vi "ExX4CamerasSameGraph.vi"() -> ()   [LabVIEW 2010]
panel:
  out "Camera 16":sgl[](graph)
  out "Camera 15":sgl[](graph)
  out "Camera 14":sgl[](graph)
  out "Camera 13":sgl[](graph)
  out "Camera 12":sgl[](graph)
  out "Camera 11":sgl[](graph)
  out "Camera 10":sgl[](graph)
  out "Camera 9":sgl[](graph)
  out "Camera 8":sgl[](graph)
  out "Camera 7":sgl[](graph)
  out "Camera 6":sgl[](graph)
  out "Camera 5":sgl[](graph)
  out "Camera 4":sgl[](graph)
  out "Camera 3":sgl[](graph)
  out "Camera 2":sgl[](graph)
  out "Camera 1":sgl[](graph)
  in  "stop":bool
  in  "Exposure":dbl=0.5 format="%.2f"
  out "error out":errorcluster
  in  "error in (no error)":errorcluster
  # "Ex2CamerasSameGraph:\nThis example runs two cameras in focus mode.\nSets them up for center strip and displays as graph.\nRemember to setup two cameras in the pvcam.ini\nfile."
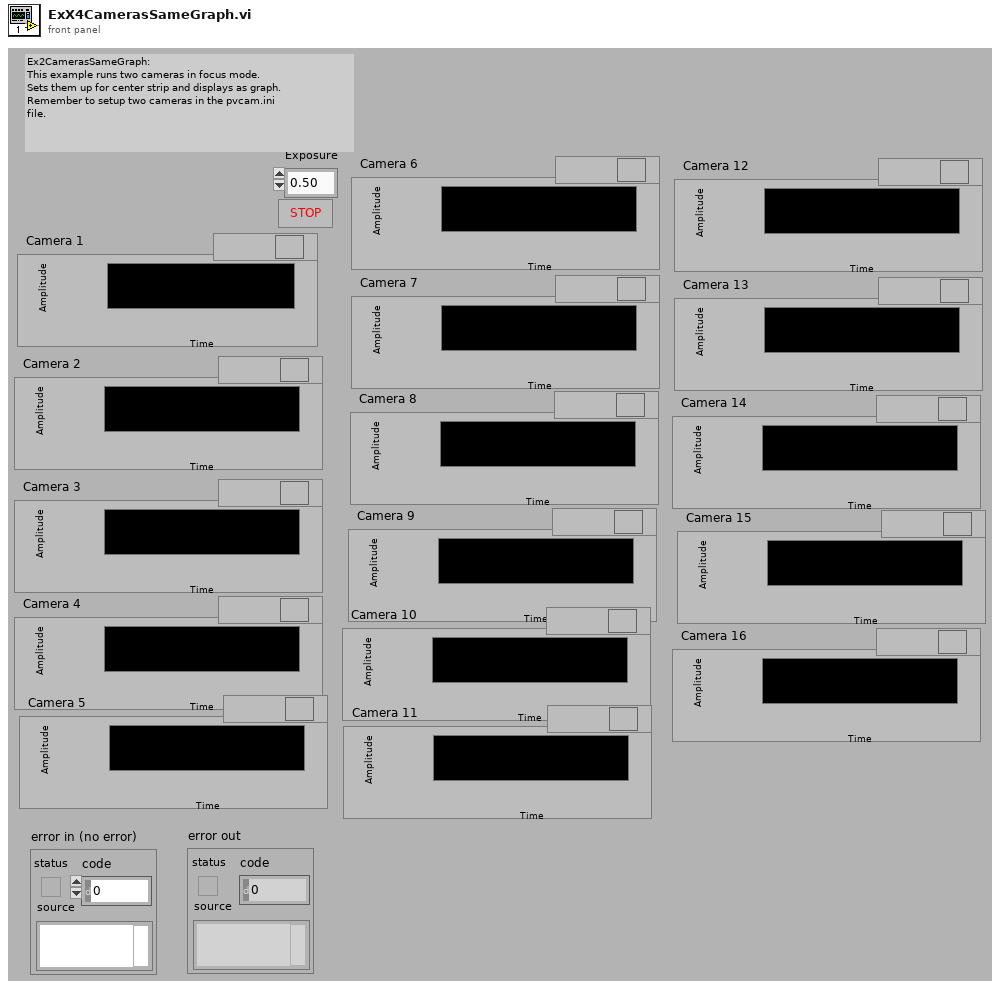
[diagram p1: front panel]
types:
  T1 = cluster{"Camera Handle":u32, "Camera Handle":u32, "Camera Handle":u32, "Camera Handle":u32}
  T2 = cluster{"Image Handle":u32, "Image Handle":u32, "Image Handle":u32, "Image Handle":u32}
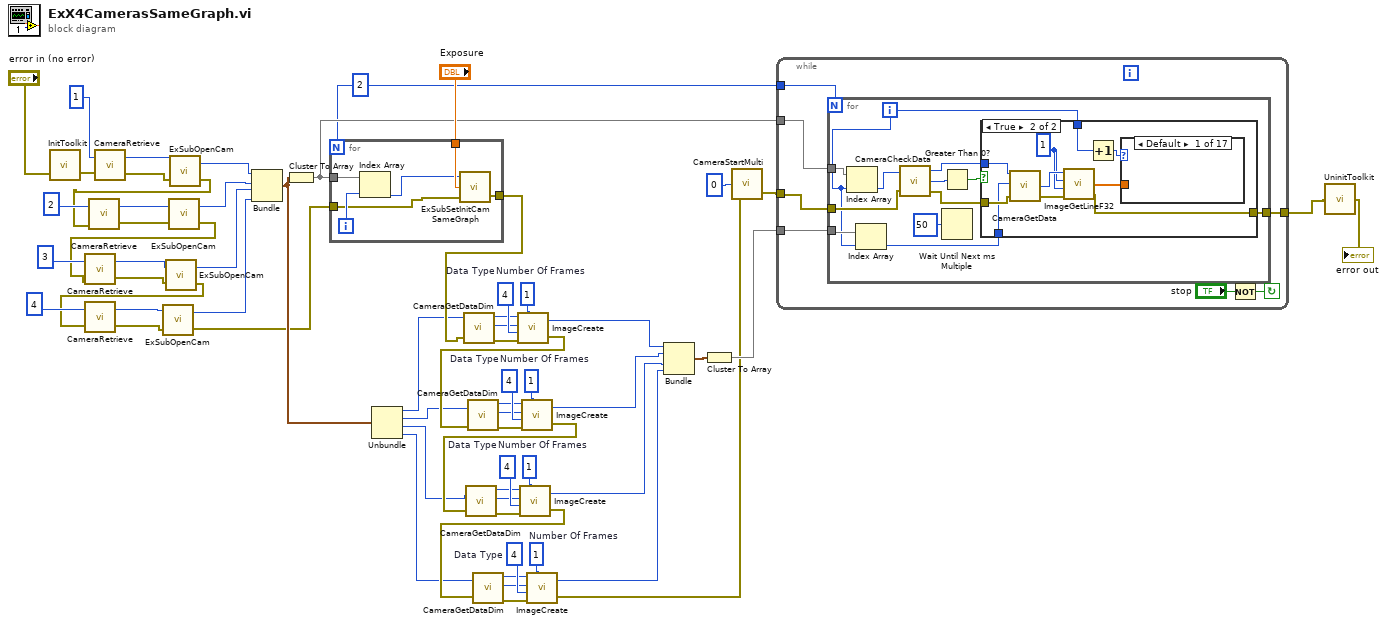
[diagram p0: block diagram]
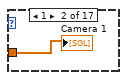
[diagram p3: hidden frame]
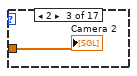
[diagram p4: hidden frame]
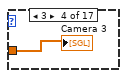
[diagram p5: hidden frame]
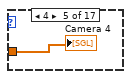
[diagram p6: hidden frame]
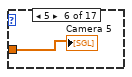
[diagram p7: hidden frame]
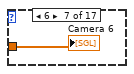
[diagram p8: hidden frame]
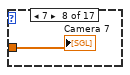
[diagram p9: hidden frame]
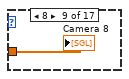
[diagram p10: hidden frame]
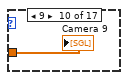
[diagram p11: hidden frame]
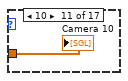
[diagram p12: hidden frame]
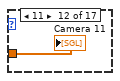
[diagram p13: hidden frame]
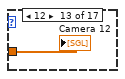
[diagram p14: hidden frame]
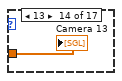
[diagram p15: hidden frame]
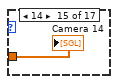
[diagram p16: hidden frame]
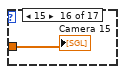
[diagram p17: hidden frame]
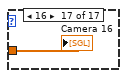
[diagram p18: hidden frame]
diagram:
  w37 = u32 1  # Number Of Frames
  w38 = u32 4  # Data Type
  w42 = u32 1  # Number Of Frames
  w43 = u32 4  # Data Type
  w47 = u32 1  # Number Of Frames
  w48 = u32 4  # Data Type
  w52 = u32 1  # Number Of Frames
  w53 = u32 4  # Data Type
  w55 = 2
  n1 = call <userlib>:"InitToolkit.vi"("error in"="error in (no error)") -> ("error out"=w64:errorcluster)
  n2 = call <userlib>:"CameraRetrieve.vi"("error in"=w64, "Camera Index"=1) -> ("error out"=w7:errorcluster, "Device ID"=w8:u32)
  n3 = call "ExSubOpenCam.vi"("error in (no error)"=w7, "Camera Device ID"=w8) -> ("error out"=w6:errorcluster, "Camera Handle"=w9:u32)
  n4 = call <userlib>:"CameraRetrieve.vi"("error in"=w6, "Camera Index"=2) -> ("error out"=w5:errorcluster, "Device ID"=w14:u32)
  n5 = call "ExSubOpenCam.vi"("error in (no error)"=w5, "Camera Device ID"=w14) -> ("error out"=w4:errorcluster, "Camera Handle"=w10:u32)
  n6 = call <userlib>:"CameraRetrieve.vi"("error in"=w4, "Camera Index"=3) -> ("error out"=w34:errorcluster, "Device ID"=w31:u32)
  n7 = call "ExSubOpenCam.vi"("error in (no error)"=w34, "Camera Device ID"=w31) -> ("error out"=w3:errorcluster, "Camera Handle"=w11:u32)
  n8 = call <userlib>:"CameraRetrieve.vi"("error in"=w3, "Camera Index"=4) -> ("error out"=w1:errorcluster, "Device ID"=w2:u32)
  n9 = call "ExSubOpenCam.vi"("error in (no error)"=w1, "Camera Device ID"=w2) -> ("error out"=w13:errorcluster, "Camera Handle"=w12:u32)
  n10 = Bundle("Camera Handle"=w9, "Camera Handle"=w10, "Camera Handle"=w11, "Camera Handle"=w12) -> (w19:T1)  [unwired: 1 in]
  n11 = Cluster To Array(cluster=w19) -> (array=w58:u32[])
  n12 = for {
    N: w55 -> [_]
    tunnel: w58 -> [w71]
    tunnel: w13 -> [w67]
    tunnel: [w69] -> w24
    tunnel: "Exposure" -> [w68]
    i -> [w70]
    n13 = Index Array(array=w71, index=w70) -> (element=w66:u32)
    n14 = call "ExSubSetInitCamSameGraph.vi"("error in (no error)"=w67, "Exposure"=w68, "Camera Handle"=w66) -> ("error out"=w69:errorcluster)  [unwired: 1 out]
  }
  n15 = Unbundle(w19) -> ("Camera Handle"=w18:u32, "Camera Handle"=w17:u32, "Camera Handle"=w16:u32, "Camera Handle"=w15:u32)
  n16 = call <userlib>:"CameraGetDataDim.vi"("Camera Handle"=w18, "error in"=w24) -> ("Xdim"=w50:u32, "Ydim"=w51:u32, "error out"=w54:errorcluster)  [unwired: 1 out]
  n17 = call <userlib>:"ImageCreate.vi"("X dimension"=w50, "Y dimension"=w51, "Data Type"=w53, "error in"=w54, "Number Of Frames"=w52) -> ("Image Handle"=w30:u32, "error out"=w23:errorcluster)
  n18 = call <userlib>:"CameraGetDataDim.vi"("Camera Handle"=w17, "error in"=w23) -> ("Xdim"=w45:u32, "Ydim"=w46:u32, "error out"=w49:errorcluster)  [unwired: 1 out]
  n19 = call <userlib>:"ImageCreate.vi"("X dimension"=w45, "Y dimension"=w46, "Data Type"=w48, "error in"=w49, "Number Of Frames"=w47) -> ("Image Handle"=w29:u32, "error out"=w22:errorcluster)
  n20 = call <userlib>:"CameraGetDataDim.vi"("Camera Handle"=w16, "error in"=w22) -> ("Xdim"=w40:u32, "Ydim"=w41:u32, "error out"=w44:errorcluster)  [unwired: 1 out]
  n21 = call <userlib>:"ImageCreate.vi"("X dimension"=w40, "Y dimension"=w41, "Data Type"=w43, "error in"=w44, "Number Of Frames"=w42) -> ("Image Handle"=w28:u32, "error out"=w21:errorcluster)
  n22 = call <userlib>:"CameraGetDataDim.vi"("Camera Handle"=w15, "error in"=w21) -> ("Xdim"=w35:u32, "Ydim"=w36:u32, "error out"=w39:errorcluster)  [unwired: 1 out]
  n23 = call <userlib>:"ImageCreate.vi"("X dimension"=w35, "Y dimension"=w36, "Data Type"=w38, "error in"=w39, "Number Of Frames"=w37) -> ("Image Handle"=w27:u32, "error out"=w20:errorcluster)
  n24 = Bundle("Image Handle"=w30, "Image Handle"=w29, "Image Handle"=w28, "Image Handle"=w27) -> (w26:T2)  [unwired: 1 in]
  n25 = Cluster To Array(cluster=w26) -> (array=w25:u32[])
  n26 = call "CameraStartMulti.vi"("error in (no error)"=w20, "Number Of Cameras"=0) -> ("error out"=w60:errorcluster)  [unwired: 1 in, 1 out]
  n27 = while {
    tunnel: w60 -> [w75]
    tunnel: w58 -> [w76]
    tunnel: [w74] -> w56
    tunnel: w55 -> [w73]
    tunnel: w25 -> [w72]
    stop <- w77 continue-if-true
    n28 = for {
      N: w73 -> [_]
      tunnel: [w85] -> w74
      tunnel: w76 -> [w84]
      tunnel: w75 -> [w82]
      tunnel: w72 -> [w81]
      i -> [w79]
      n29 = Index Array(array=w84, index=w79) -> (element=w83:u32)
      n30 = Index Array(array=w81, index=w79) -> (element=w80:u32)
      n31 = call <userlib>:"CameraCheckData.vi"("Camera Handle"=w83, "error in"=w82) -> ("Camera Handle"=w87:u32, "Number Of Frames Available"=w89:i32, "error out"=w86:errorcluster)
      n32 = Greater Than 0?(x=w89) -> (x > 0?=w88:bool)
      n33 = Wait Until Next ms Multiple(millisecond multiple=u32 50) -> ()  [unwired: 1 out]
      n34 = case shown="True" w88 {
        tunnel: [w91 w98] -> w85
        tunnel: w87 -> [_ w97]
        tunnel: w86 -> [w91 w96]
        tunnel: w79 -> [_ w92]
        tunnel: w80 -> [_ w94]
        frame False {
        }
        frame True {
          w99 = 1
          n35 = call <userlib>:"CameraGetData.vi"("error in"=w96, "Data Handle"=w94, "Camera Handle"=w97) -> ("error out"=w101:errorcluster, "Data Handle"=w100:u32)  [unwired: 1 out]
          n36 = call <userlib>:"ImageGetLineF32.vi"("error in"=w101, "Z Position"=w99, "Y Position"=w99, "Data Handle"=w100) -> ("error out"=w98:errorcluster, "Array F32"=w95:sgl[])  [unwired: 1 out]
          n37 = Increment(x=w92) -> (x+1=w93:i32)
          n38 = case shown="Default" w93 {
            tunnel: w95 -> [_ w102 w103 w104 w105 w106 w107 w108 w109 w110 w111 w112 w113 w114 w115 w116 w117]
            frame Default {
            }
            frame 1 {
              "Camera 1" <- w102
            }
            frame 2 {
              "Camera 2" <- w103
            }
            frame 3 {
              "Camera 3" <- w104
            }
            frame 4 {
              "Camera 4" <- w105
            }
            frame 5 {
              "Camera 5" <- w106
            }
            frame 6 {
              "Camera 6" <- w107
            }
            frame 7 {
              "Camera 7" <- w108
            }
            frame 8 {
              "Camera 8" <- w109
            }
            frame 9 {
              "Camera 9" <- w110
            }
            frame 10 {
              "Camera 10" <- w111
            }
            frame 11 {
              "Camera 11" <- w112
            }
            frame 12 {
              "Camera 12" <- w113
            }
            frame 13 {
              "Camera 13" <- w114
            }
            frame 14 {
              "Camera 14" <- w115
            }
            frame 15 {
              "Camera 15" <- w116
            }
            frame 16 {
              "Camera 16" <- w117
            }
          }
        }
      }
    }
    n39 = Not(x="stop") -> (.not. x?=w77:bool)
  }
  n40 = call <userlib>:"UninitToolkit.vi"("error in"=w56) -> ("error out"=→"error out":errorcluster)
